vi "Pre-existing Assert.vi"(8 "error in (no error)":errorcluster, 10 "UID String":string, 11 "Standard Display Configuration in":refnum<class "Standard Display Configuration.lvclass">) -> (0 "error out":errorcluster, 1 "Assert Index":i32, 2 "Assert Name":string, 3 "Assert Exists":bool)   [LabVIEW 2016, in "Assert API Components.lvlib" / "Assert Display.lvlib" / "Main Display.lvlib" / "Standard Display Configuration.lvclass"]
uses:
  Standard Display Configuration.lvclass
  C:/Users/ukhornp/Documents/Work/Projects/actor_assert_api/Core/Main Display/Display Configurations/Base Display Configuration.lvclass
  Base Display Configuration.lvclass/Base Display Configuration.ctl
  Base Display Configuration.lvclass
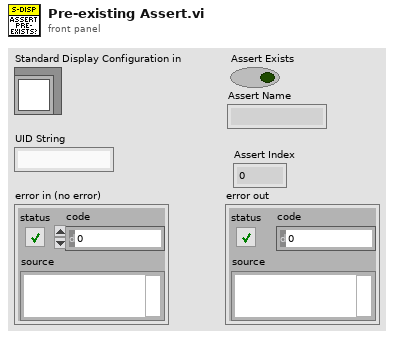
[diagram p1: front panel]
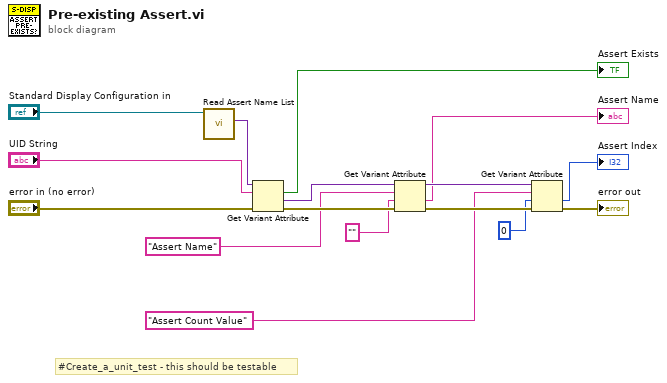
[diagram p0: block diagram]
diagram:
  # "#Create_a_unit_test - this should be testable"
  n1 = call "Read Assert Name List.vi"("Base Display Configuration in"="Standard Display Configuration in") -> ("Assert Name List"=w13:variant)  [unwired: 10 in]
  n2 = Get Variant Attribute(Variant=w13, name="UID String", error in="error in (no error)") -> (found=→"Assert Exists":bool, value=w7:variant, error out=w12:errorcluster)  [unwired: 1 in, 1 out]
  n3 = Get Variant Attribute(Variant=w7, name="Assert Name", default value (empty Variant)="", error in=w12) -> (duplicate Variant=w8:variant, value=→"Assert Name":string, error out=w10:errorcluster)  [unwired: 1 out]
  n4 = Get Variant Attribute(Variant=w8, name="Assert Count Value", default value (empty Variant)=0 ("Assert Index"), error in=w10) -> (value=→"Assert Index":i32, error out=→"error out":errorcluster)  [unwired: 2 out]
